vi "Read value from ini file.vi"(10 "Section":string="ProductID", 11 "Ini file name":string="Toggle 8 defaults.ini") -> (2 "Values":string[](array[string]), 3 "Key names":string[](array[string]))   [LabVIEW 2020]
uses:
  <vilib>/Utility/config.llb/Read Key (String).vi
  <vilib>/Utility/config.llb/NI_LVConfig.lvlib
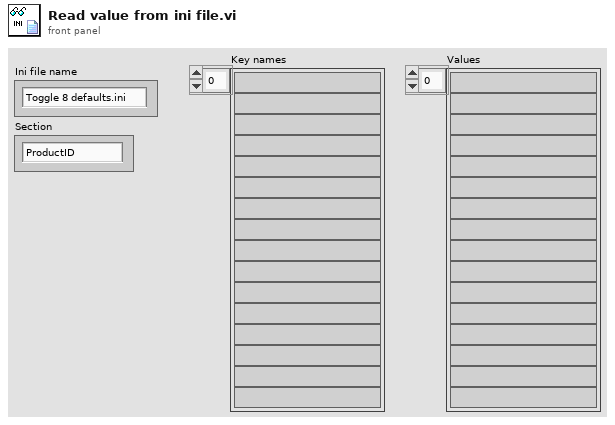
[diagram p1: front panel]
types:
  T1 = typedef "NI_LVConfig.lvlib/Config Data RefNum.ctl" = refnum<k1>
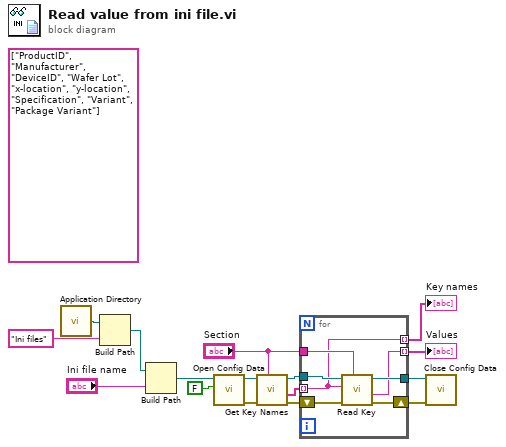
[diagram p0: block diagram]
diagram:
  (unwired) string[] ["ProductID", "Manufacturer", "DeviceID", "Wafer Lot", "x-location", "y-location", "Specification", "Variant", "Package Variant"]
  n1 = call <vilib>:"Application Directory.vi"() -> ("Application Directory"=w16:path)
  n2 = Build Path(base path=w16, name or relative path="Ini files") -> (appended path=w7:path)
  n3 = Build Path(base path=w7, name or relative path="Ini file name") -> (appended path=w13:path)
  n4 = call <vilib>:"Open Config Data.vi"("create file if necessary (T)"=FALSE, "configuration file path"=w13) -> ("error out"=w11:errorcluster, "refnum"=w10:T1)  [unwired: 7 in, 1 out]
  n5 = call <vilib>:"Get Key Names.vi"("section"="Section", "error in (no error)"=w11, "refnum"=w10) -> ("error out"=w4:errorcluster, "key names"=w2:string[], "refnum out"=w3:T1)  [unwired: 5 in, 1 out]
  n6 = for {
    tunnel: w3 -> [w23]
    tunnel: w2 -> [w17] mode=indexing
    tunnel: "Section" -> [w21]
    shift-right: [w20] -> w9
    shift-left: w4 -> [w22]
    tunnel: [w19] -> w8
    tunnel: [w18] -> w6 mode=indexing
    tunnel: [w17] -> w1 mode=indexing
    n7 = call-poly <vilib>:"Read Key.vi"("section"=w21, "error in (no error)"=w22, "key"=w17, "refnum"=w23) -> ("error out"=w20:errorcluster, "value"=w18:string, "refnum out"=w19:T1)  [unwired: 4 in, 1 out]
  }
  "Values" <- w6
  "Key names" <- w1
  n8 = call <vilib>:"Close Config Data.vi"("error in (no error)"=w9, "refnum"=w8) -> ()  [unwired: 8 in, 2 out]
